vi "specu1a 1.0.0 TD Clean.vi"(3 "type string in":i16[](array[numeric]) format="%.0x") -> (0 "Cleaned Type String out":i16[](array[numeric]) format="%.0x", 1 "Type string out":i16[](array[numeric]) format="%.0x")   [LabVIEW 2010]
uses:
  Controls/specu1a 1.0.0 TD Data type.ctl
panel:
  out "Array":T1[](array[typedef]) format="%.0x"
  in  "Data type":T1 format="%.0x"
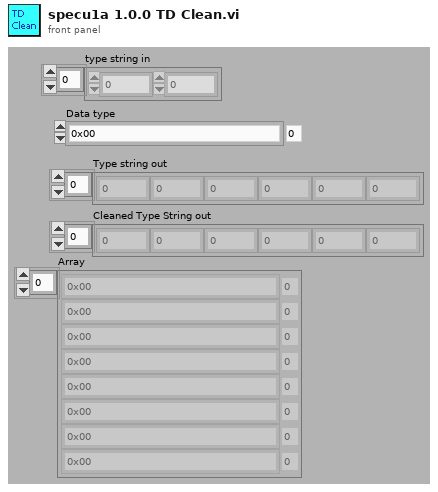
[diagram p1: front panel]
types:
  T1 = typedef "specu1a 1.0.0 TD Data type.ctl" = enum8{"0x00", "0x01 Byte Integer", "0x02 Word Integer", "0x03 Long Integer", "0x04", "0x05 Unsigned Byte Integer", "0x06 Unsigned Word Integer", "0x07 Unsigned Long Integer", "0x08", "0x09 SGL Floating Point Number", "0x0A DBL Floating Point Number", "0x0B EXT Floating Point Number", "0x0C SGL Complex Number", "0x0D DBL Complex Number", "0x0E EXT Complex Number", "0x0F", "0x10", "0x11", "0x12", "0x13", "0x14", "0x15 Enum Byte Integer", "0x16 Enum Word Integer", "0x17 Enum Long Integer", "0x18", "0x19 SGL Float Physical Quantity", "0x1A DBL Float Physical Quantity", "0x1B EXT Float Physical Quantity", "0x1C SGL Complex Physical Quantity", "0x1D DBL Complex Physical Quantity", "0x1E EXT Complex Physical Quantity", "0x1F", "0x20", "0x21 Boolean", "0x22", "0x23", "0x24", "0x25", "0x26", "0x27", "0x28", "0x29", "0x2A", "0x2B", "0x2C", "0x2D", "0x2E", "0x2F", "0x30 String", "0x31", "0x32 Path", "0x33 Pict", "0x34", "0x35", "0x36", "0x37 DAQ", "0x38", "0x39", "0x3A", "0x3B", "0x3C", "0x3D", "0x3E", "0x3F", "0x40 Array", "0x41", "0x42", "0x43", "0x44", "0x45", "0x46", "0x47", "0x48", "0x49", "0x4A", "0x4B", "0x4C", "0x4D", "0x4E", "0x4F", "0x50 Cluster", "0x51", "0x52", "0x53 Variant", "0x54", "0x55", "0x56", "0x57", "0x58", "0x59", "0x5A", "0x5B", "0x5C", "0x5D", "0x5E", "0x5F", "0x60", "0x61", "0x62", "0x63", "0x64", "0x65", "0x66", "0x67", "0x68", "0x69", "0x6A", "0x6B", "0x6C", "0x6D", "0x6E", "0x6F", "0x70 Refnum (VISA etc.)"}
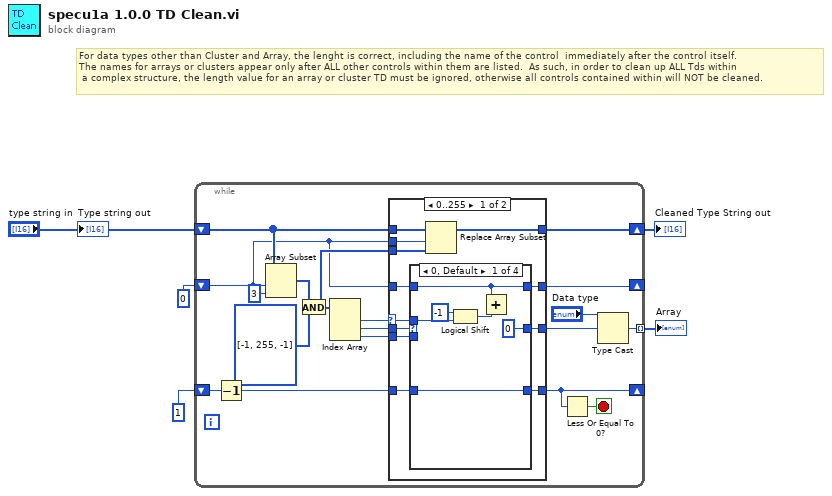
[diagram p0: block diagram]
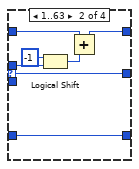
[diagram p2: hidden frame]
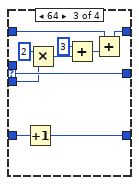
[diagram p3: hidden frame]
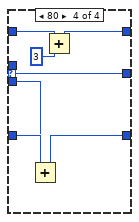
[diagram p4: hidden frame]
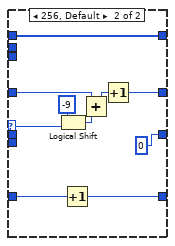
[diagram p5: hidden frame]
diagram:
  # "For data types other than Cluster and Array, the lenght is correct, including the name of the control  immediately after the control itself.\nThe names for arrays or clusters appear only after ALL other controls within them are listed.  As such, in order to clean up ALL Tds within\n a complex structure, the length value for an array or cluster TD must be ignored, otherwise all controls contained within will NOT be cleaned."
  n1 = while {
    shift-right: [w10] -> w3
    shift-left: "type string in" -> [w13]
    shift-right: [w6] -> _
    shift-left: 0 -> [w11]
    tunnel: [w18] -> w2 mode=indexing
    shift-right: [w14] -> _
    shift-left: 1 -> [w17]
    stop <- w15 stop-if-true
    n2 = Decrement(x=w17) -> (x-1=w16:i32)
    n3 = Array Subset(array=w13, index=w11, length=3) -> (w22:i16[])
    n4 = And(x=w22, y=i16[] [-1, 255, -1] ("*(type *) &x 2")) -> (x .and. y?=w12:i16[])
    n5 = Index Array(array=w12) -> (element #1=w7:i16, element #2=w8:i16, element #3=w9:i16)  [unwired: 3 in]
    n6 = case shown="0..255" w7 {
      selector: w7 -> [w24 w66]
      tunnel: w11 -> [w35 w75]
      tunnel: [w34 i16 0] -> w19
      tunnel: w9 -> [w33 _]
      tunnel: w8 -> [w32 _]
      tunnel: w16 -> [w31 w74]
      tunnel: [w30 w67] -> w6
      tunnel: [w29 w73] -> w14
      tunnel: w13 -> [w28 w71]
      tunnel: w12 -> [w27 _]
      tunnel: w11 -> [w26 _]
      tunnel: [w25 w71] -> w10
      frame 0..255 {
        n7 = case shown="0, Default" w32 {
          selector: w32 -> [_ w48 w53 w65]
          tunnel: [u16 0 w48 w53 w65] -> w34
          tunnel: w35 -> [w39 w45 w57 w63]
          tunnel: [w39 w47 w56 w62] -> w30
          tunnel: w24 -> [w37 w43 _ _]
          tunnel: w33 -> [_ _ w51 w60]
          tunnel: w31 -> [w40 w46 w55 w61]
          tunnel: [w40 w46 w54 w59] -> w29
          frame 0, Default {
            n8 = Logical Shift(y=-1, x=w37) -> (x << y=w36:i16)
            n9 = Add(x=w39, y=w36) -> ()  [unwired: 1 out]
          }
          frame 1..63 {
            n10 = Logical Shift(y=-1, x=w43) -> (x << y=w42:i16)
            n11 = Add(x=w45, y=w42) -> (x+y=w47:i32)
          }
          frame 64 {
            n12 = Increment(x=w55) -> (x+1=w54:i32)
            n13 = Multiply(x=2, y=w51) -> (x*y=w49:i32)
            n14 = Add(x=3, y=w49) -> (x+y=w58:i32)
            n15 = Add(x=w57, y=w58) -> (x+y=w56:i32)
          }
          frame 80 {
            n16 = Add(x=w60, y=w61) -> (x+y=w59:i32)
            n17 = Add(x=w63, y=3) -> (x+y=w62:i32)
          }
        }
        n18 = Replace Array Subset(array=w28, new element=w27, index=w26) -> (w25:i16[])
      }
      frame 256, Default {
        n19 = Logical Shift(y=-9, x=w66) -> (x << y=w68:i16)
        n20 = Increment(x=w74) -> (x+1=w73:i32)
        n21 = Add(x=w75, y=w68) -> (x+y=w70:i32)
        n22 = Increment(x=w70) -> (x+1=w67:i32)
      }
    }
    n23 = Less Or Equal To 0?(x=w14) -> (x <= 0?=w15:bool)
    n24 = Type Cast(type="Data type", x=w19) -> (*(type *) &x=w18:T1)
  }
  "Cleaned Type String out" <- w3
  "Array" <- w2
  "Type string out" <- "type string in"
